vi "Scale Ort Data.vi"(10 "Pitch (Arg 2)":string, 11 "Roll (Arg 3)":string) -> (2 "Latitude":dbl, 3 "Longitude":dbl)   [LabVIEW 2014]
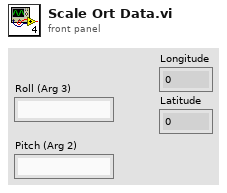
[diagram p1: front panel]
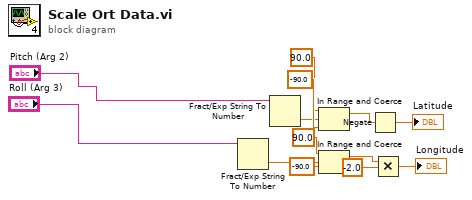
[diagram p0: block diagram]
diagram:
  n1 = Fract/Exp String To Number(string="Roll (Arg 3)") -> (number=w5:dbl)  [unwired: 3 in, 1 out]
  n2 = Fract/Exp String To Number(string="Pitch (Arg 2)") -> (number=w3:dbl)  [unwired: 3 in, 1 out]
  n3 = In Range and Coerce(upper limit=90.0, x=w3, lower limit=-90.0) -> (coerced(x)=w13:dbl)  [unwired: 1 out]
  n4 = In Range and Coerce(upper limit=90.0, x=w5, lower limit=-90.0) -> (coerced(x)=w11:dbl)  [unwired: 1 out]
  n5 = Negate(x=w13) -> (-x=→"Latitude":dbl)
  n6 = Multiply(x=w11, y=-2.0) -> (x*y=→"Longitude":dbl)
